vi "Baratron Pressure.vi"(8 "error in (no error)":errorcluster, 10 "Baratron Pressure":waveform(dbl), 11 "Baratron Pressure in":refnum<class "Baratron Pressure.lvclass">) -> (0 "error out":errorcluster, 3 "Baratron Pressure out":refnum<class "Baratron Pressure.lvclass">)   [LabVIEW 2021, in "Baratron Pressure.lvlib" / "Baratron Pressure.lvclass"]
uses:
  Baratron Pressure.lvclass
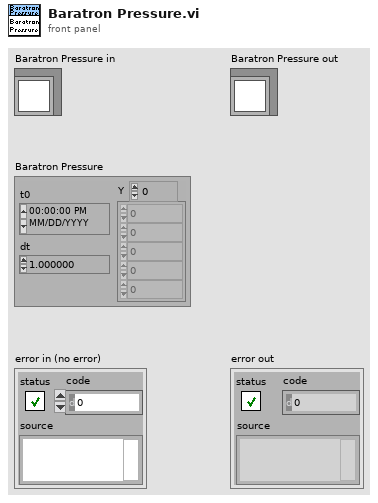
[diagram p1: front panel]
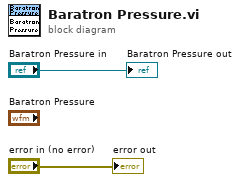
[diagram p0: block diagram]
diagram:
  "error out" <- "error in (no error)"
  "Baratron Pressure out" <- "Baratron Pressure in"
